vi "Opg1.vi"() -> ()   [LabVIEW 2022 SP3]
uses:
  <vilib>/Utility/error.llb/DialogType.ctl
  <vilib>/DAQmx/write.llb/DAQmx Write (Digital 1D Bool NChan 1Samp 1Line).vi
  <vilib>/DAQmx/read.llb/DAQmx Read.vi
  <vilib>/DAQmx/read.llb/DAQmx Read (Analog 1D DBL NChan 1Samp).vi
  <vilib>/DAQmx/write.llb/DAQmx Write (Counter Frequency 1Chan 1Samp).vi
  <extravilib>/ChannelInstances/Tag-dbl/Write With Abort.vi
  <extravilib>/ChannelInstances/Tag-dbl/Read With Abort.vi
  <vilib>/DAQmx/create/channels.llb/DAQmx Create Channel (CO-Pulse Generation-Frequency).vi
  <vilib>/DAQmx/configure/timing.llb/DAQmx Timing (Implicit).vi
  <extravilib>/ChannelInstances/Tag-dbl/Instantiate.vi
  <extravilib>/ChannelInstances/Tag-dbl/EndpointRead.vi
  <vilib>/DAQmx/miscellaneous.llb/DAQmx Fill In Error Info.vi
  <extravilib>/ChannelInstances/Tag-dbl/Endpoint.vi
  <extravilib>/ChannelInstances/Tag-dbl.lvlib
panel:
  in  "Kd":dbl
  out "Temp":dbl
  in  "Ki":dbl
  out "x+y":dbl
  out "data":dbl[](array[numeric]) format="%#_6p"
  out "element":dbl
  in  "KP":dbl
  in  "SetPunkt":dbl
  in  "Frekvens":dbl=100.0 caption="Frequency (Hz)" format="%0.2f"
  in  "Counter(s)":tag="myDAQ1/ctr0" caption="PWM Counter(s)"
  in  "stop 2":bool caption="stop"
  in  "Boolean":bool
  out "Waveform Chart":dbl(graph)
  in  "stop":bool
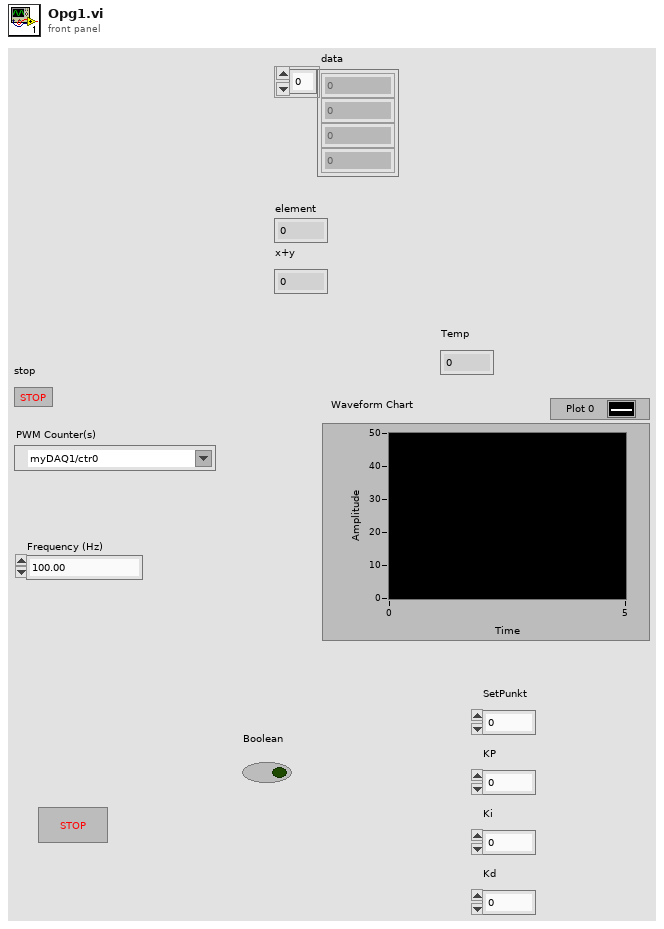
[diagram p1: front panel]
types:
  T1 = typedef "DialogType.ctl" = u16
  T2 = typedef "Tag-dbl.lvlib/))Channel.ctl" = refnum<queue>
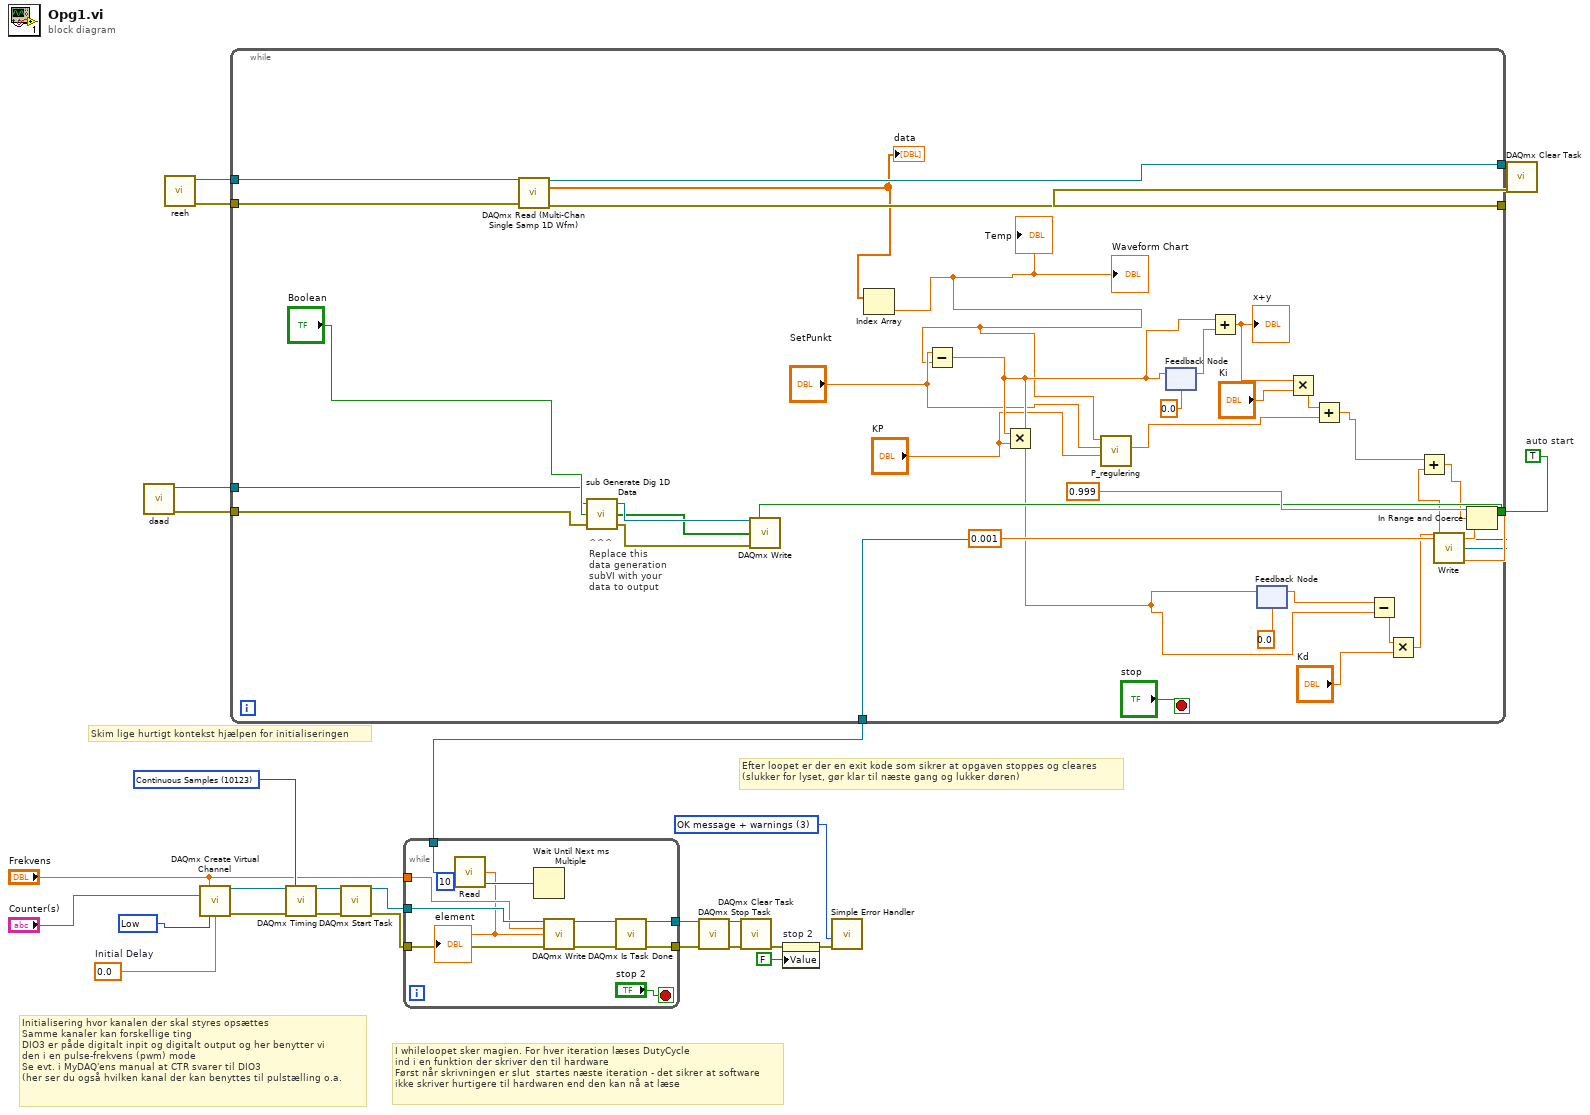
[diagram p0: block diagram]
diagram:
  w1 = TRUE  # auto start
  w17 = 0.0  # Initial Delay
  w19 = 10214 items=["High"=10192, "Low"=10214] ("Idle State")
  w18 = T1 3 items=["no dialog", "OK message", "continue or stop message", "OK message + warnings", "continue/stop + warnings"] ("type of dialog (OK msg:1)")
  w21 = 10123 items=["Finite Samples"=10178, "Continuous Samples"=10123] ("sample mode")
  # "Efter loopet er der en exit kode som sikrer at opgaven stoppes og cleares\n(slukker for lyset, gør klar til næste gang og lukker døren)"
  # "I whileloopet sker magien. For hver iteration læses DutyCycle\nind i en funktion der skriver den til hardware\nFørst når skrivningen er slut  startes næste iteration - det sikrer at software\nikke skriver hurtigere til hardwaren end den kan nå at læse"
  # "Skim lige hurtigt kontekst hjælpen for initialiseringen"
  # "Initialisering hvor kanalen der skal styres opsættes\nSamme kanaler kan forskellige ting\nDIO3 er påde digitalt inpit og digitalt output og her benytter vi \nden i en pulse-frekvens (pwm) mode\nSe evt. i MyDAQ'ens manual at CTR svarer til DIO3\n(her ser du også hvilken kanal der kan benyttes til pulstælling o.a."
  n1 = call "daad.vi"() -> ("error out"=w3:errorcluster, "task out"=w2:refnum<k21>)  [unwired: 10 in]
  n2 = call "reeh.vi"() -> ("error out"=w5:errorcluster, "task out"=w4:refnum<k21>)  [unwired: 10 in]
  n3 = call-poly <vilib>:"DAQmx Create Virtual Channel.vi"("frequency"="Frekvens", "counter"="Counter(s)", "idle state"=w19, "initial delay"=w17) -> ("task out"=w25:refnum<k21>, "error out"=w27:errorcluster)  [unwired: 10 in]
  n4 = while {
    tunnel: [w57] -> w8
    tunnel: [w56] -> w7
    tunnel: [w55] -> w6
    tunnel: w5 -> [w54]
    tunnel: w4 -> [w53]
    tunnel: w3 -> [w51]
    tunnel: w2 -> [w50]
    tunnel: w1 -> [w48]
    stop <- "stop" stop-if-true
    # "^^^\nReplace this\ndata generation\nsubVI with your\ndata to output"
    n5 = call-poly "DAQmx Read (Multi-Chan Single Samp 1D Wfm).vi"("task/channels in"=w53, "error in"=w54) -> ("task out"=w56:refnum<k21>, "data"=w43:dbl[], "error out"=w55:errorcluster)  [unwired: 11 in]
    "data" <- w43
    n6 = call <vilib>:"sub Generate Dig 1D Data.vi"("error in"=w51, "initial value"="Boolean", "task in"=w50) -> ("error out"=w46:errorcluster, "Data"=w47:bool[], "task out"=w49:refnum<k21>)
    n7 = call-poly <vilib>:"DAQmx Write.vi"("task/channels in"=w49, "auto start"=w48, "data"=w47, "error in"=w46) -> ()  [unwired: 9 in, 3 out]
    n8 = Index Array(array=w43) -> (element=w28:dbl)  [unwired: 1 in]
    "Waveform Chart" <- w28
    "Temp" <- w28
    n9 = Subtract(x="SetPunkt", y=w28) -> (x-y=w37:dbl)
    n10 = Multiply(x=w37, y="KP") -> ()  [unwired: 1 out]
    n11 = call "P_regulering.vi"("k_p"="KP", "SP"="SetPunkt", "DATA"=w28) -> ("e(t)"=w31:dbl)  [unwired: 7 in, 1 out]
    n12 = feedback-in #1(w37) -> ()
    n13 = feedback #1(0.0) -> (w44:dbl)
    n14 = Add(x=w37, y=w44) -> (x+y=w42:dbl)
    "x+y" <- w42
    n15 = feedback-in #2(w37) -> ()
    n16 = feedback #2(0.0) -> (w38:dbl)
    n17 = Multiply(x=w42, y="Ki") -> (x*y=w40:dbl)
    n18 = Add(x=w40, y=w31) -> (x+y=w34:dbl)
    n19 = Subtract(x=w38, y=w37) -> (x-y=w35:dbl)
    n20 = Multiply(x=w35, y="Kd") -> (x*y=w33:dbl)
    n21 = Add(x=w34, y=w33) -> (x+y=w32:dbl)
    n22 = In Range and Coerce(upper limit=0.999, x=w32, lower limit=0.001) -> (coerced(x)=w58:dbl)  [unwired: 1 out]
    n23 = call <extravilib>:"Write.vi"("element"=w58) -> ("channel"=w57:T2)  [unwired: 1 out]
  }
  n24 = call-poly <vilib>:"DAQmx Timing.vi"("task/channels in"=w25, "sample mode"=w21, "error in"=w27) -> ("task out"=w22:refnum<k21>, "error out"=w23:errorcluster)  [unwired: 11 in]
  n25 = call <vilib>:"DAQmx Start Task.vi"("task/channels in"=w22, "error in"=w23) -> ("task out"=w24:refnum<k21>, "error out"=w26:errorcluster)  [unwired: 12 in]
  n26 = while {
    tunnel: w26 -> [w66]
    tunnel: w24 -> [w67]
    tunnel: [w72] -> w12
    tunnel: [w71] -> w10
    tunnel: "Frekvens" -> [w65]
    tunnel: w8 -> [w63]
    stop <- "stop 2" stop-if-true
    n27 = call <extravilib>:"Read.vi"("channel"=w63) -> ("element"=w62:dbl)  [unwired: 1 in, 1 out]
    "element" <- w62
    n28 = Wait Until Next ms Multiple(millisecond multiple=u32 10) -> ()  [unwired: 1 out]
    n29 = call-poly <vilib>:"DAQmx Write.vi"("task/channels in"=w67, "frequency"=w65, "duty cycle"=w62, "error in"=w66) -> ("task out"=w69:refnum<k21>, "error out"=w68:errorcluster)  [unwired: 9 in, 1 out]
    n30 = call <vilib>:"DAQmx Is Task Done.vi"("task/channels in"=w69, "error in"=w68) -> ("task out"=w72:refnum<k21>, "error out"=w71:errorcluster)  [unwired: 11 in, 1 out]
  }
  n31 = call <vilib>:"DAQmx Stop Task.vi"("task/channels in"=w12, "error in"=w10) -> ("task out"=w11:refnum<k21>, "error out"=w9:errorcluster)  [unwired: 12 in]
  n32 = call <vilib>:"DAQmx Clear Task.vi"("task in"=w11, "error in"=w9) -> ("error out"=w13:errorcluster)  [unwired: 13 in]
  n33 = property on="stop 2" class="Bool (strict)"(error in=w13, "Value"=FALSE ("stop")) -> (error out=w14:errorcluster)  [unwired: 1 in, 1 out]
  n34 = call <vilib>:"Simple Error Handler.vi"("type of dialog (OK msg:1)"=w18, "error in (no error)"=w14) -> ()  [unwired: 3 in, 5 out]
  n35 = call <vilib>:"DAQmx Clear Task.vi"("task in"=w7, "error in"=w6) -> ()  [unwired: 13 in, 1 out]
